vi "Export Data.vi"() -> ()   [LabVIEW 2020]
panel:
  out "data":string[][](array[string])
  in  "Export":bool
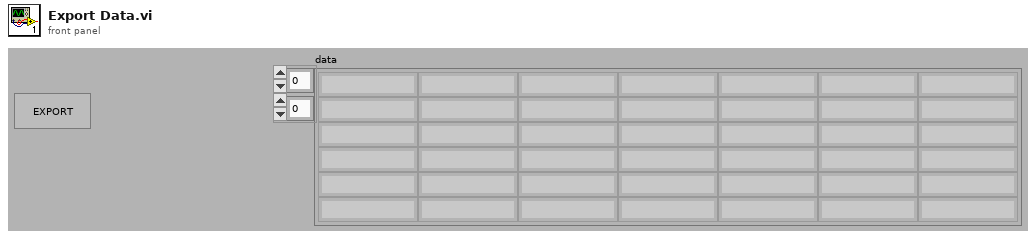
[diagram p1: front panel]
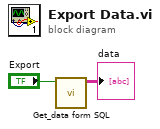
[diagram p0: block diagram]
diagram:
  n1 = call "Get_data form SQL.vi"("Export"="Export") -> ("data"=→"data":string[][])  [unwired: 9 in, 1 out]
